vi "Update power status.vi"(10 "SystemPowerStatus in":T2, 11 "UPS status in":T1 {"Last update" format="%<%H:%M:%S>T"}) -> (0 "error out":errorcluster, 2 "UPS status out":T1 {"Last update" format="%<%H:%M:%S>T"}, 3 "SystemPowerStatus out":T2)   [LabVIEW 2024, in "Power monitor.lvlib"]
uses:
  Power monitor.lvlib
  C:/Windows/System32/kernel32.dll
  .net PowerModeChanged/dotNET PowerModeChanged.llb/SystemPowerStatus.ctl
  PwrM status.ctl
panel:
  in  "Visa name":refnum<visa-resource-name>="COM5"
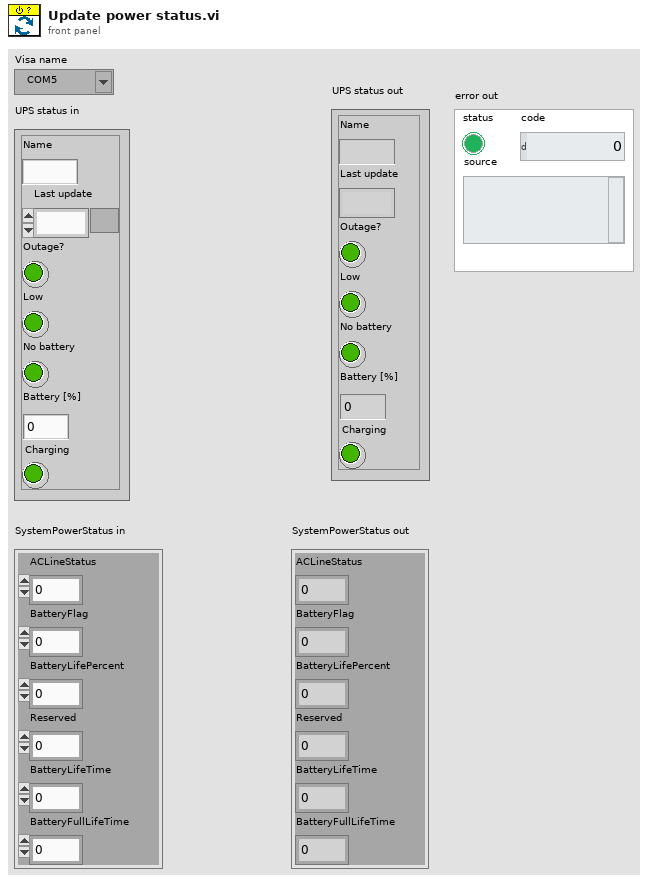
[diagram p1: front panel]
types:
  T1 = typedef "Power monitor.lvlib/PwrM status.ctl" = cluster{"Name":string, "Last update":timestamp, "Outage?":bool, "Low":bool, "No battery":bool, "Battery [%]":u8, "Charging":bool}
  T2 = typedef "SystemPowerStatus.ctl" = cluster{"ACLineStatus":u8, "BatteryFlag":u8, "BatteryLifePercent":u8, "Reserved":u8, "BatteryLifeTime":i32, "BatteryFullLifeTime":i32}
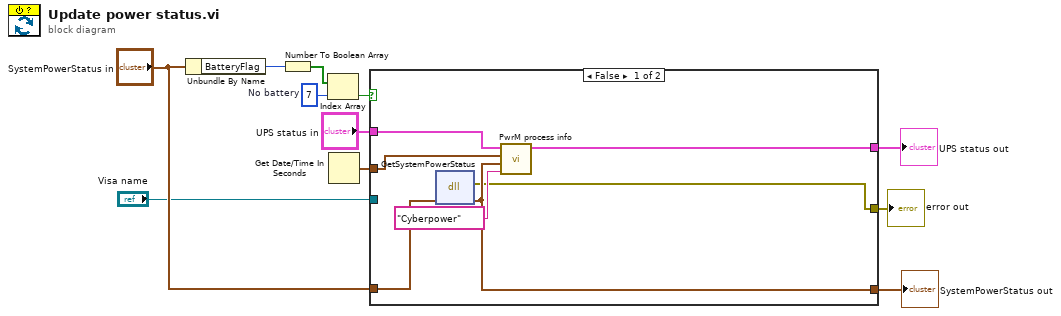
[diagram p0: block diagram]
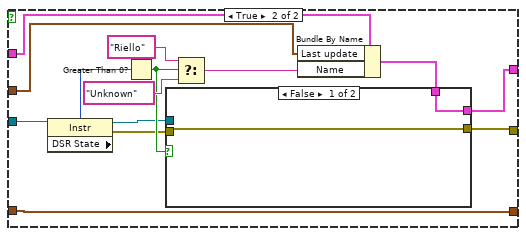
[diagram p2: hidden frame]
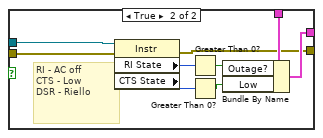
[diagram p3: hidden frame]
diagram:
  w3 = 7  # No battery
  n1 = Unbundle By Name("SystemPowerStatus in") -> ("BatteryFlag"=w4:u8)
  n2 = Number To Boolean Array(number=w4) -> (Boolean array=w6:bool[])
  n3 = Index Array(array=w6, index=w3) -> (element=w5:bool)
  n4 = Get Date/Time In Seconds() -> (seconds since 1Jan1904=w8:timestamp)
  n5 = case shown="False" w5 {
    tunnel: "UPS status in" -> [w17 w32]
    tunnel: [w18 w23] -> w9
    tunnel: w8 -> [w16 w31]
    tunnel: "SystemPowerStatus in" -> [w14 w30]
    tunnel: [w13 w30] -> w11
    tunnel: "Visa name" -> [_ w21]
    tunnel: [w12 w19] -> w1
    frame False {
      n6 = dll-call lib="C:/Windows/System32/kernel32.dll" fn="GetSystemPowerStatus"("PWR info cluster"=w14) -> (error out=w12:errorcluster, "PWR info cluster"=w13:T2)  [unwired: 4 in, 1 out]
      n7 = call "PwrM process info.vi"("Name"="Cyberpower", "PWR info cluster"=w13, "Timestamp"=w16, "UPS in"=w17) -> ("UPS out"=w18:T1)  [unwired: 7 in]
    }
    frame True {
      n8 = property class="Instr"(reference=w21) -> (reference out=w22:refnum<visa-resource-name>, error out=w20:errorcluster, "DSR State"=w29:i16)  [unwired: 1 in]
      n9 = Greater Than 0?(x=w29) -> (x > 0?=w25:bool)
      n10 = Select(t="Riello" ("Name"), s=w25, f="Unknown" ("Name")) -> (s? t:f=w26:string)
      n11 = Bundle By Name(cluster=w32, "Last update"=w31, "Name"=w26) -> (w24:T1)
      n12 = case shown="False" w25 {
        tunnel: w24 -> [w34 w43]
        tunnel: [w34 w42] -> w23
        tunnel: w22 -> [_ w37]
        tunnel: w20 -> [w33 w36]
        tunnel: [w33 w35] -> w19
        frame False {
        }
        frame True {
          # "RI - AC off\nCTS - Low \nDSR - Riello"
          n13 = property class="Instr"(reference=w37, error in=w36) -> (error out=w35:errorcluster, "RI State"=w41:i16, "CTS State"=w40:i16)  [unwired: 1 out]
          n14 = Greater Than 0?(x=w41) -> (x > 0?=w39:bool)
          n15 = Greater Than 0?(x=w40) -> (x > 0?=w38:bool)
          n16 = Bundle By Name(cluster=w43, "Outage?"=w39, "Low"=w38) -> (w42:T1)
        }
      }
    }
  }
  "SystemPowerStatus out" <- w11
  "UPS status out" <- w9
  "error out" <- w1
